vi "Configure External Data Log Trigger Source.vi"(8 "error in (no error)":errorcluster {"code" format="%.0x"}, 9 "External Logger Trigger Source (0: Bus)":i32(ring) items=["Bus", "External", "Immediate", "Pin 1", "Pin 2", "Pin 3", "Pin 4", "Pin 5", "Pin 6", "Pin 7"], 10 "Channel Name (1)":string="1", 11 "VISA resource name":refnum<visa-resource-name>) -> (0 "error out":errorcluster {"code" format="%.0x"}, 3 "VISA resource name out":refnum<visa-resource-name>)   [LabVIEW 2018, in "Agilent N6700 Series.lvlib"]
doc: "Configures the trigger source for the external data logger."
uses:
  Agilent N6700 Series.lvlib
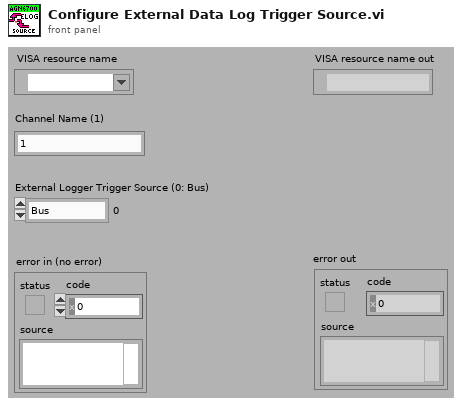
[diagram p1: front panel]
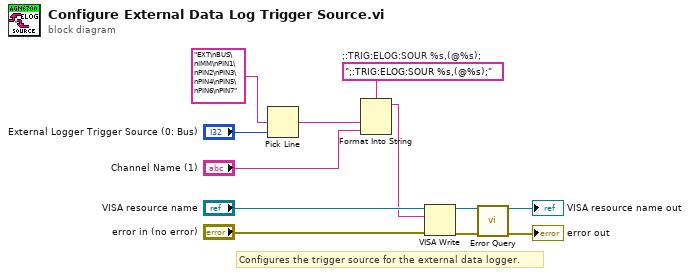
[diagram p0: block diagram]
diagram:
  w12 = ";:TRIG:ELOG:SOUR %s,(@%s);"  # ;:TRIG:ELOG:SOUR %s,(@%s);
  # "Configures the trigger source for the external data logger."
  n1 = Pick Line(multi-line string="EXT\nBUS\nIMM\nPIN1\nPIN2\nPIN3\nPIN4\nPIN5\nPIN6\nPIN7", line index="External Logger Trigger Source (0: Bus)") -> (output string=w8:string)  [unwired: 1 in]
  n2 = Format Into String(format string=w12, w8, "Channel Name (1)") -> (resulting string=w6:string)  [unwired: 2 in, 1 out]
  n3 = VISA Write(VISA resource name="VISA resource name", write buffer=w6, error in (no error)="error in (no error)") -> (VISA resource name out=w2:refnum<visa-resource-name>, error out=w1:errorcluster)  [unwired: 1 out]
  n4 = call "Error Query.vi"("VISA resource name"=w2, "error in (no error)"=w1) -> ("VISA resource name out"=→"VISA resource name out":refnum<visa-resource-name>, "error out"=→"error out":errorcluster)  [unwired: 10 in, 2 out]
